vi "Write alive_.vi"(8 "error in (no error)":errorcluster, 10 "alive?":bool, 11 "Human in":refnum<class "Human.lvclass">) -> (0 "error out":errorcluster, 3 "Human out":refnum<class "Human.lvclass">)   [LabVIEW 2019, in "Human.lvclass"]
uses:
  Human.lvclass
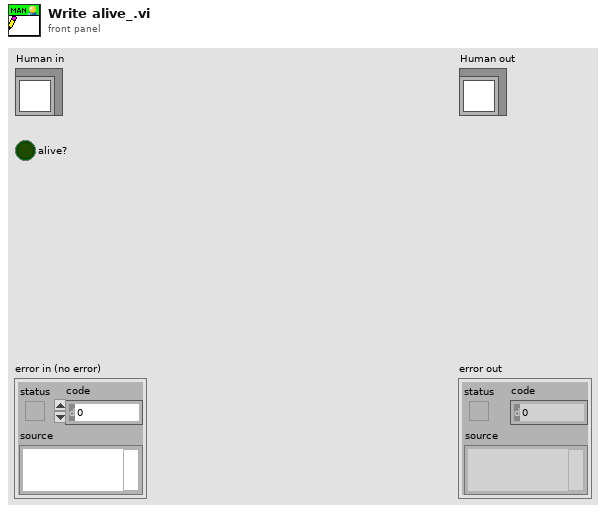
[diagram p1: front panel]
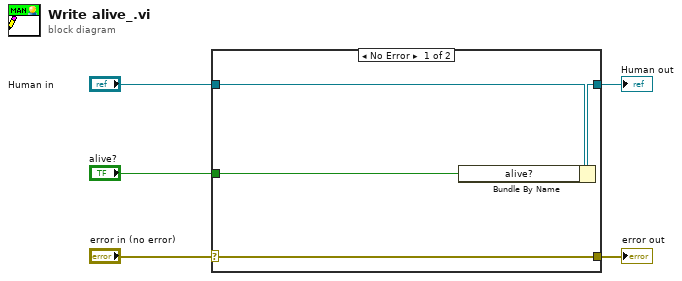
[diagram p0: block diagram]
diagram:
  n1 = case shown="No Error" "error in (no error)" {
    selector: "error in (no error)" -> [w9 w10]
    tunnel: [w9 w10] -> w4
    tunnel: [w7 w11] -> w2
    tunnel: "Human in" -> [w8 w11]
    tunnel: "alive?" -> [w6 _]
    frame No Error {
      n2 = Bundle By Name(cluster=w8, "alive?"=w6) -> (w7:refnum<class "Human.lvclass">)
    }
    frame Error {
    }
  }
  "error out" <- w4
  "Human out" <- w2
